vi "SysLog Status Filtern.vi"(11 "Message Array":string[](array[string])) -> (3 "Message Array":string[](array[string]))   [LabVIEW 2020, in "SysLog.lvlib"]
doc: "PasswortLevel für die Anzeige des SysLog berücksichtigen - für das Statusfenster ..."
uses:
  SysLog.lvlib
  Passwortverwaltung/FGV Passwort Aktion.ctl
  SysLogSort.ctl
  Passwortverwaltung/Passwort.lvlib
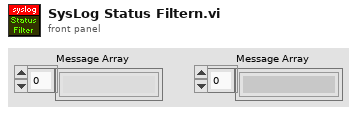
[diagram p1: front panel]
types:
  T1 = typedef "Passwort.lvlib/FGV Passwort Aktion.ctl" = enum16{"prüfen", "setzen", "Initialisieren", "PW speichern", "lesen", "PW Änderung"}
  T2 = typedef "SysLog.lvlib/SysLogSort.ctl" = cluster{"interne":enum16{"alle", "nur benutzerrelevante", "nur interne"}, "Typ":enum16{"*", "Err+Warn", "Err", "Warn", "OK"}, "Sortierung":enum16{"Zeit", "Code", "Typ"}, "Richtung":enum16{"v", "^"}, "Filter":string}
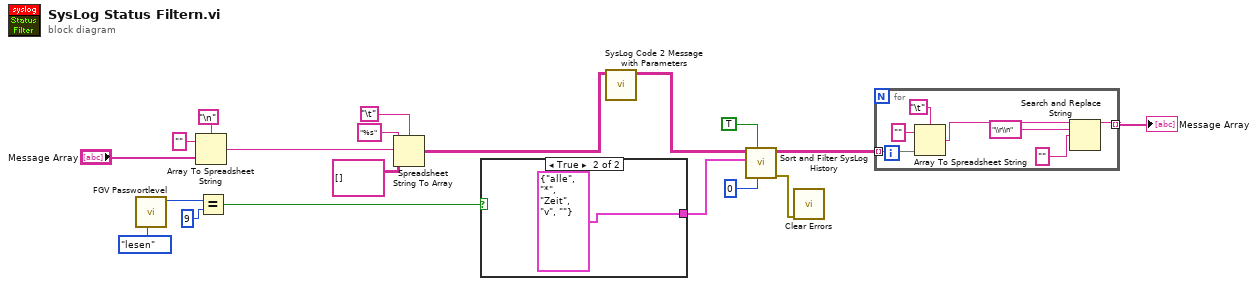
[diagram p0: block diagram]
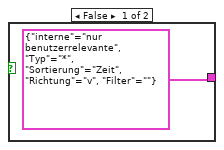
[diagram p2: hidden frame]
diagram:
  n1 = call "FGV Passwortlevel.vi"("FGV Passwort Aktion"=FGV_Passwort_Aktion."lesen") -> ("aktueller Level"=w16:i16)  [unwired: 3 in, 7 out]
  n2 = Array To Spreadsheet String(delimiter (Tab)="\n", array="Message Array", 3:"" ("Format-String")) -> (spreadsheet string=w9:string)
  n3 = Equal?(x=w16, y=i16 9) -> (x = y?=w19:bool)
  n4 = Spreadsheet String To Array(delimiter (Tab)="\t", format string="%s" ("Tabellen-String"), spreadsheet string=w9, array type (2D Dbl)=string[][] [] ("Array-Typ (2D Dbl)")) -> (array=w2:string[][])
  n5 = case shown="True" w19 {
    tunnel: [T2 {"interne"=enum."nur benutzerrelevante", "Typ"=enum."*", "Sortierung"=enum."Zeit", "Richtung"=enum."v", "Filter"=""} ("Cluster (in)") T2 {"interne"=enum."alle", "Typ"=enum."*", "Sortierung"=enum."Zeit", "Richtung"=enum."v", "Filter"=""} ("Cluster (in)")] -> w8
    frame False {
    }
    frame True {
    }
  }
  n6 = call "SysLog Code 2 Message with Parameters.vi"("Array-Typ (2D Dbl) (Eingang)"=w2) -> ("Array-Typ (2D Dbl) (Ausgang)"=w1:string[][])  [unwired: 10 in]
  n7 = call "Sort and Filter SysLog History.vi"("Spaltenindex intern"=u32 0, "NoSort"=TRUE, "Cluster (in)"=w8, "Array-Typ (2D Dbl) in"=w1) -> ("Fehler (out)"=w7:errorcluster, "Array-Typ (2D Dbl) out"=w6:string[][])  [unwired: 6 in]
  n8 = call <vilib>:"Clear Errors.vi"("error in (no error)"=w7) -> ()  [unwired: 5 in, 2 out]
  n9 = for {
    tunnel: w6 -> [w27] mode=indexing
    tunnel: [w24] -> w5 mode=indexing
    n10 = Array To Spreadsheet String(delimiter (Tab)="\t", array=w27, 3:"" ("Format-String")) -> (spreadsheet string=w25:string)
    n11 = Search and Replace String(input string=w25, search string="\\r\\n", replace string="" ("Format-String")) -> (result string=w24:string)  [unwired: 5 in, 3 out]
  }
  "Message Array" <- w5
